vi "Read y.vi"(8 "error in (no error)":errorcluster, 11 "Diamond in":refnum<class "Diamond.lvclass">) -> (0 "error out":errorcluster, 2 "y":dbl[](array[numeric]), 3 "Diamond out":refnum<class "Diamond.lvclass">)   [LabVIEW 2021, in "d15.lvlib" / "Diamond.lvclass"]
uses:
  Diamond.lvclass
  Diamond.lvclass/Diamond.ctl
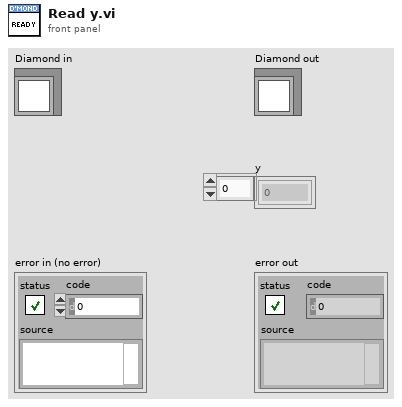
[diagram p1: front panel]
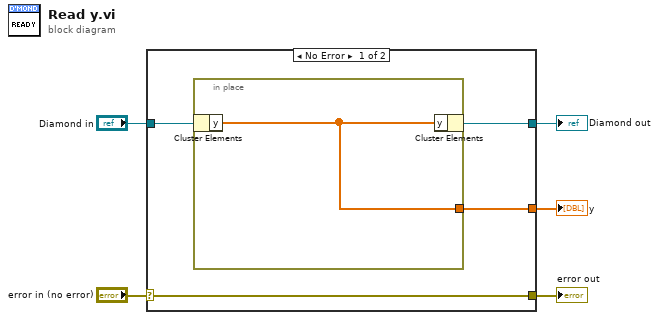
[diagram p0: block diagram]
diagram:
  n1 = case shown="No Error" "error in (no error)" {
    selector: "error in (no error)" -> [w9 w11]
    tunnel: [w9 w11] -> w4
    tunnel: [w6 w12] -> w2
    tunnel: "Diamond in" -> [w7 w12]
    tunnel: [w8 _] -> w1
    frame No Error {
      n2 = in-place {
        in-place-border: [w10] -> w8
        n3 = in-place-cluster #1(w7) -> ("y"=w10:dbl[])
        n4 = in-place-cluster #1("y"=w10) -> (w6:refnum<class "Diamond.lvclass">)
      }
    }
    frame Error {
    }
  }
  "error out" <- w4
  "Diamond out" <- w2
  "y" <- w1
